vi "Test Missing Libraries.vi"(11 "Test Case In":refnum<class "Missing in Project.lvclass">) -> (0 "error out":errorcluster, 3 "Test Case Out":refnum<class "Missing in Project.lvclass">)   [LabVIEW 2021, in "Missing in Project.lvclass"]
doc: "Tests to make sure all libraries defined in the project are saved to disk."
uses:
  Missing in Project.lvclass
  C:/Program Files/National Instruments/LabVIEW 2024/vi.lib/Astemes/LUnit/Test Case.lvclass
  <vilib>/Astemes/LUnit/Test Case.lvclass/Test Case.ctl
  <vilib>/Astemes/LUnit/Core/LUnit Test Case/Private/Append Pass Result.vi
  <vilib>/Astemes/LUnit/Core/LUnit Test Case/Private/Append Fail Result.vi
  <vilib>/Astemes/LUnit/Core/LUnit Test Case/Private/Run In UI.vi
  <vilib>/Utility/error.llb/Clear Errors.vi
  <vilib>/Astemes/LUnit/Test Case.lvclass
panel:
  out "Missing items from LabVIEW project":path[](array[path])
  out "Pass":bool
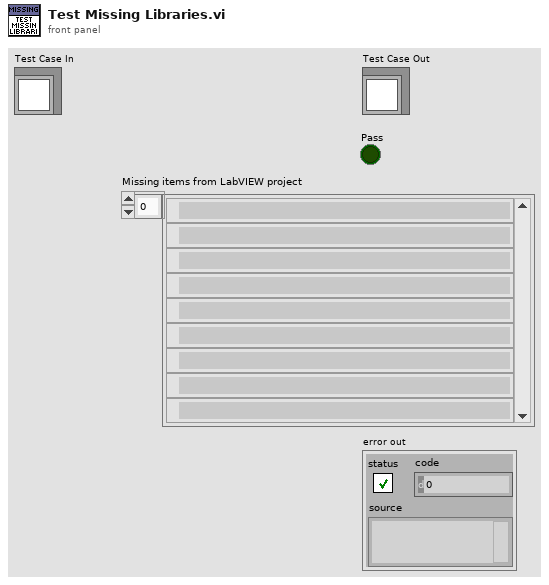
[diagram p1: front panel]
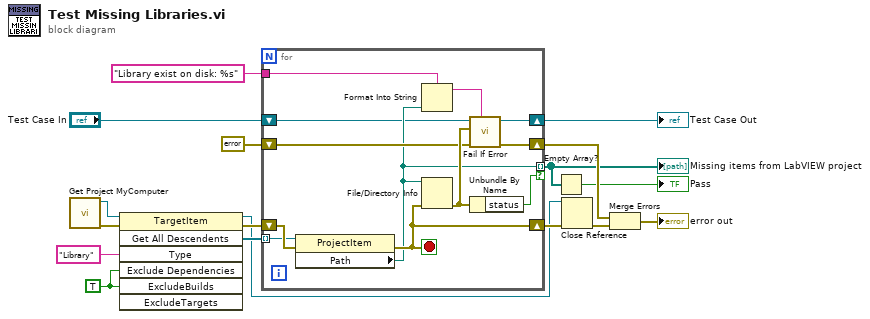
[diagram p0: block diagram]
diagram:
  w1 = TRUE ("ExcludeBuilds")
  n1 = call "Get Project MyComputer.vi"() -> ("error out"=w13:errorcluster, "My Computer"=w5:refnum<vi>)  [unwired: 10 in]
  n2 = invoke class="TargetItem" method="Get All Descendents"(reference=w5, error in=w13, "Type"="Library", "Exclude Dependencies"=w1, "ExcludeBuilds"=w1) -> (reference out=w8:refnum<vi>, error out=w17:errorcluster, "All Descendents"=w9:refnum<vi>[])  [unwired: 2 in, 4 out]
  n3 = for {
    tunnel: w9 -> [w24] mode=indexing
    shift-right: [w27] -> w16
    shift-left: w17 -> [w28]
    tunnel: [w23] -> w6 mode=indexing if=w20
    shift-right: [w25] -> w11
    shift-left: errorcluster {"status"=FALSE, "code"=0, "source"=""} ("error in (no error)") -> [w26]
    shift-right: [w22] -> w3
    shift-left: "Test Case In" -> [w21]
    tunnel: "Library exist on disk: %s" ("Label") -> [w19]
    stop <- w27 stop-if-true
    n4 = property class="ProjectItem"(reference=w24, error in=w28) -> (error out=w27:errorcluster, "Path"=w23:path)  [unwired: 1 out]
    n5 = Format Into String(format string=w19, w23) -> (resulting string=w18:string)  [unwired: 2 in, 1 out]
    n6 = File/Directory Info(path=w23, error in=w27) -> (error out=w29:errorcluster)  [unwired: 6 out]
    n7 = call <vilib>:"Fail If Error.vi"("Description"=w18, "error in (no error)"=w26, "Assert error"=w29, "LUnit Test Case In"=w21) -> ("error out"=w25:errorcluster, "LUnit Test Case Out"=w22:refnum<class "Missing in Project.lvclass">)  [unwired: 6 in]
    n8 = Unbundle By Name(w29) -> ("status"=w20:bool)
  }
  "Missing items from LabVIEW project" <- w6
  "Test Case Out" <- w3
  n9 = Empty Array?(array=w6) -> (empty?=→"Pass":bool)
  n10 = Close Reference(reference=w8, error in (no error)=w16) -> (error out=w15:errorcluster)
  n11 = Merge Errors(w11, w15) -> (→"error out":errorcluster)
